vi "FacadeResizable2DArray(String).vi"(0 "Data In":T4, 2 "Display State In":T2, 3 "Container State":T3) -> (6 "Data Out":T4, 7 "Display State Out":T2, 8 "Action":T1)   [LabVIEW 2011, in "Resizable2DArray(String).xctl"]
uses:
  <vilib>/_probes/SAPHIR/ViBox - Probes/Resizable2DArray/Resizable2DArray(String)/Resizable2DArray(String).xctl
  <vilib>/_probes/SAPHIR/ViBox - Probes/Resizable2DArray/Resizable2DArray(String)/DataResizable2DArray(String).ctl
  <vilib>/_xctls/Container State.ctl
  <vilib>/_probes/SAPHIR/ViBox - Probes/Resizable2DArray/Resizable2DArray(String)/StateResizable2DArray(String).ctl
  <vilib>/_xctls/Action.ctl
  <vilib>/_xctls/XControlSupport.lvlib
panel:
  in  "DisplayFormat":enum16{"Normal", "Code", "Hex"}(ring) caption="Display format :"
  out "String":string
  out "[Strings]":string[][](array[string])
  # "Display Options"
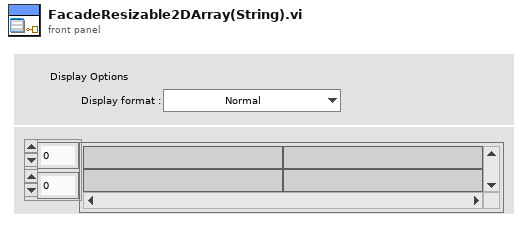
[diagram p1: front panel]
types:
  T1 = typedef "XControlSupport.lvlib/Action.ctl" = cluster{"Data Changed?":bool, "State Changed?":bool, "Action Name":string}
  T2 = typedef "Resizable2DArray(String).xctl/StateResizable2DArray(String).ctl" = cluster{"Height":u32, "Width":u32}
  T3 = typedef "XControlSupport.lvlib/Container State.ctl" = cluster{"Indicator?":bool, "Run Mode?":bool, " Refnum":refnum<vi>}
  T4 = typedef "Resizable2DArray(String).xctl/DataResizable2DArray(String).ctl" = string[][]
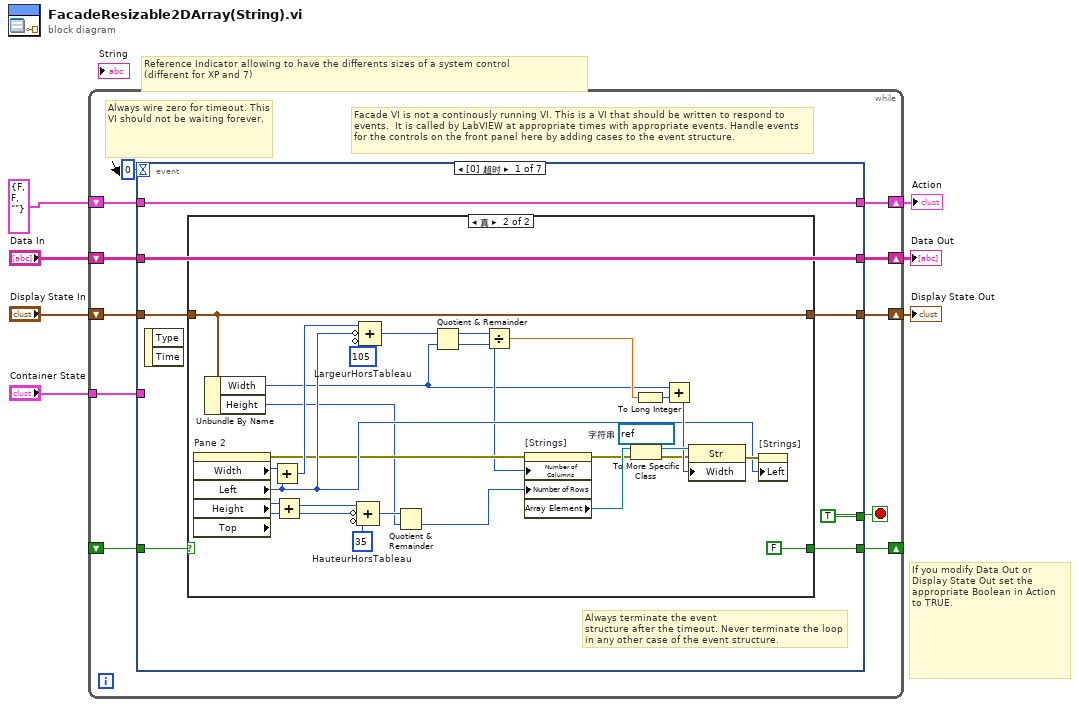
[diagram p0: block diagram]
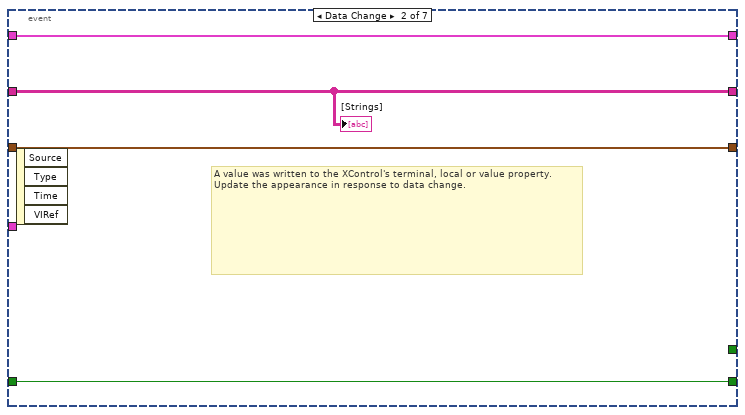
[diagram p3: hidden frame]
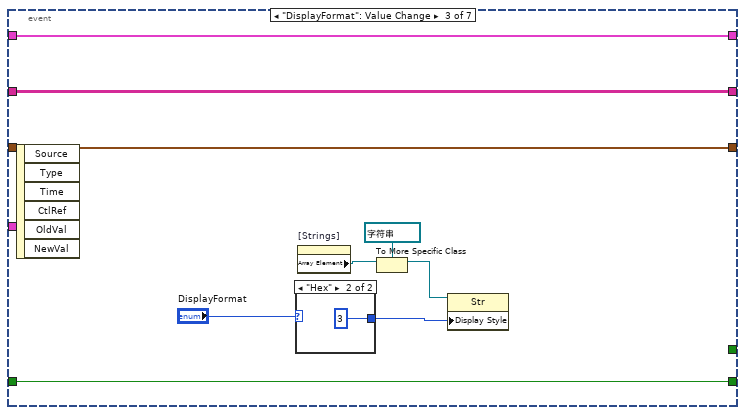
[diagram p4: hidden frame]
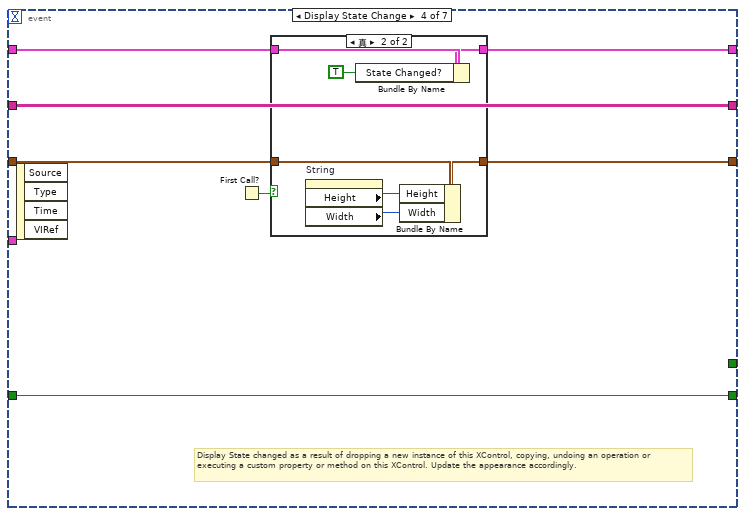
[diagram p6: hidden frame]
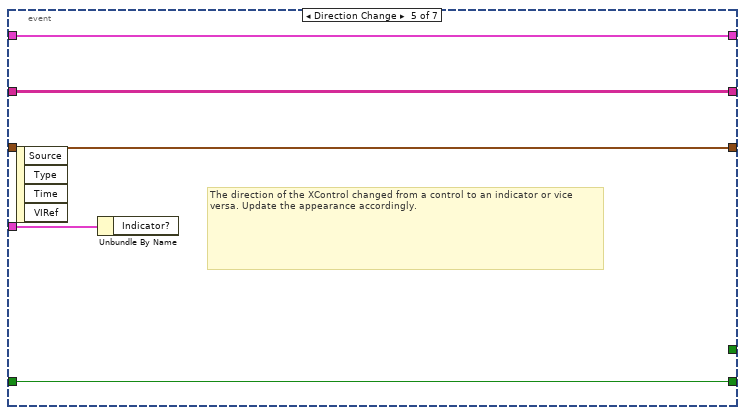
[diagram p8: hidden frame]
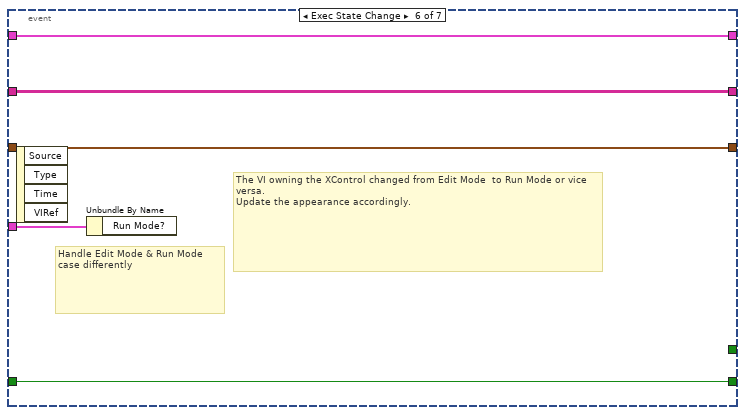
[diagram p9: hidden frame]
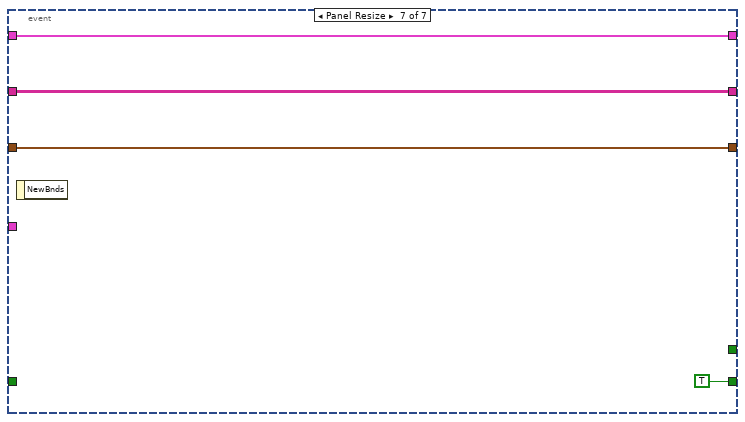
[diagram p10: hidden frame]
diagram:
  # "Reference Indicator allowing to have the differents sizes of a system control\n(different for XP and 7)"
  # "If you modify Data Out or\nDisplay State Out set the\nappropriate Boolean in Action\nto TRUE."
  n1 = while {
    shift-right: [w17] -> w5
    shift-left: "Display State In" -> [w18]
    tunnel: "Container State" -> [w14]
    shift-right: [w12] -> w7
    shift-left: "Data In" -> [w13]
    shift-right: [w10] -> w3
    shift-left: T1 {"Data Changed?"=FALSE, "State Changed?"=FALSE, "Action Name"=""} ("Action") -> [w11]
    shift-right: [w8] -> _
    shift-left: _ -> [w9]
    stop <- w16 stop-if-true
    # "Facade VI is not a continously running VI. This is a VI that should be written to respond to events.  It is called by LabVIEW at appropriate times with appropriate events. Handle events for the controls on the front panel here by adding cases to the event structure."
    # "Always wire zero for timeout. This\nVI should not be waiting forever."
    n2 = event shown="[0] 超时" {
      selector: _ -> [_ _ _ _ _ _ _]
      dyn-events: _ -> [_ _ _ _ _ _ _]
      timeout: 0 -> [_ _ _ _ _ _ _]
      tunnel: w18 -> [w20 w58 w67 w71 w89 w94 w98]
      tunnel: [w19 w58 w67 w70 w89 w94 w98] -> w17
      tunnel: [TRUE _ _ _ _ _ _] -> w16
      tunnel: w14 -> [_ _ _ _ w90 w95 _]
      tunnel: w13 -> [w23 w56 w66 w76 w88 w93 w99]
      tunnel: [w23 w56 w66 w76 w88 w93 w99] -> w12
      tunnel: [w24 w57 w65 w72 w87 w92 w97] -> w10
      tunnel: w11 -> [w24 w57 w65 w73 w87 w92 w97]
      tunnel: w9 -> [w22 w55 w59 w75 w86 w91 _]
      tunnel: [w21 w55 w59 w75 w86 w91 TRUE] -> w8
      event Timeout {
        # "Always terminate the event\nstructure after the timeout. Never terminate the loop in any other case of the event structure."
        n3 = event-data() -> ()  [unwired: 3 out]
        n4 = case shown="真" w22 {
          selector: w22 -> [w27 _]
          tunnel: [w27 FALSE] -> w21
          tunnel: w20 -> [w26 w30]
          tunnel: [w26 w30] -> w19
          frame False {
          }
          frame True {
            w52 = refnum<vi> refnum  # 字符串
            w54 = i16 35  # HauteurHorsTableau
            w53 = i16 105  # LargeurHorsTableau
            n5 = property on="Pane 2" class="Pane"() -> (error out=w36:errorcluster, "Width"=w38:u32, "Left"=w39:i32, "Height"=w34:u32, "Top"=w35:i32)  [unwired: 2 in, 1 out]
            n6 = Unbundle By Name(w30) -> ("Width"=w29:u32, "Height"=w28:u32)
            n7 = Add(x=w38, y=w39) -> (x+y=w40:u32)
            n8 = Add(x=w34, y=w35) -> (x+y=w37:u32)
            n9 = Compound Arithmetic op=ADD(w37, invert w35, invert w54) -> (w45:u32)
            n10 = Compound Arithmetic op=ADD(w40, invert w39, invert w53) -> (w49:u32)
            n11 = Quotient & Remainder(x=w45, y=w28) -> (floor(x/y)=w32:u32)  [unwired: 1 out]
            n12 = Quotient & Remainder(x=w49, y=w29) -> (x-y*floor(x/y)=w41:u32, floor(x/y)=w33:u32)
            n13 = Divide(x=w41, y=w33) -> (x/y=w48:dbl)
            n14 = property on="[Strings]" class="Arr (严格)"(error in=w36, "Number of Columns"=w33, "Number of Rows"=w32) -> (error out=w44:errorcluster, "Array Element"=w46:refnum<vi>)  [unwired: 1 in, 1 out]
            n15 = To More Specific Class(target class=w52, reference=w46, error in=w44) -> (specific class reference=w51:refnum<vi>, error out=w43:errorcluster)
            n16 = To Long Integer(number=w48) -> (32bit integer=w47:i32)
            n17 = Add(x=w29, y=w47) -> (x+y=w50:u32)
            n18 = property class="Str"(reference=w51, error in=w43, "Width"=w50) -> (error out=w42:errorcluster)  [unwired: 1 out]
            n19 = property on="[Strings]" class="Arr (严格)"(error in=w42, "Left"=w39) -> ()  [unwired: 1 in, 2 out]
          }
        }
      }
      event Data Change {
        # "A value was written to the XControl's terminal, local or value property.\nUpdate the appearance in response to data change."
        n20 = event-data() -> ()  [unwired: 5 out]
        "[Strings]" <- w56
      }
      event "DisplayFormat": Value Change {
        n21 = event-data() -> ()  [unwired: 7 out]
        n22 = case shown="\"Hex\"" "DisplayFormat" {
          selector: "DisplayFormat" -> [w68 _]
          tunnel: [w68 u32 3 ("Display Style")] -> w64
          frame Default {
          }
          frame "Hex" {
          }
        }
        n23 = property on="[Strings]" class="Arr (严格)"() -> ("Array Element"=w61:refnum<vi>)  [unwired: 2 in, 2 out]
        n24 = To More Specific Class(target class=refnum<vi> refnum ("specific class reference"), reference=w61) -> (specific class reference=w63:refnum<vi>)  [unwired: 1 in, 1 out]
        n25 = property class="Str"(reference=w63, "Display Style"=w64) -> ()  [unwired: 1 in, 2 out]
      }
      event Display State Change {
        # "Display State changed as a result of dropping a new instance of this XControl, copying, undoing an operation or executing a custom property or method on this XControl. Update the appearance accordingly."
        n26 = event-data() -> ()  [unwired: 5 out]
        n27 = First Call?() -> (First Call?: T/F=w74:bool)
        n28 = case shown="真" w74 {
          tunnel: w71 -> [w78 w85]
          tunnel: [w78 w84] -> w70
          tunnel: w73 -> [w77 w82]
          tunnel: [w77 w81] -> w72
          frame False {
          }
          frame True {
            n29 = property on="String" class="Str"() -> ("Height"=w83:u32, "Width"=w79:u32)  [unwired: 2 in, 2 out]
            n30 = Bundle By Name(cluster=w82, "State Changed?"=TRUE) -> (w81:T1)
            n31 = Bundle By Name(cluster=w85, "Height"=w83, "Width"=w79) -> (w84:T2)
          }
        }
      }
      event Direction Change {
        # "The direction of the XControl changed from a control to an indicator or vice versa. Update the appearance accordingly."
        n32 = event-data() -> ()  [unwired: 5 out]
        n33 = Unbundle By Name(w90) -> ()  [unwired: 1 out]
      }
      event Exec State Change {
        # "The VI owning the XControl changed from Edit Mode  to Run Mode or vice versa.\nUpdate the appearance accordingly."
        # "Handle Edit Mode & Run Mode\ncase differently"
        n34 = event-data() -> ()  [unwired: 5 out]
        n35 = Unbundle By Name(w95) -> ()  [unwired: 1 out]
      }
      event Panel Resize {
        n36 = event-data() -> ()  [unwired: 2 out]
      }
    }
  }
  "Display State Out" <- w5
  "Data Out" <- w7
  "Action" <- w3
